vi "movimientocabinas.vi"() -> ()   [LabVIEW 2021]
panel:
  in  "BB 5":bool
  out "Graficas":cluster{"CabinaA":dbl, "CabinaB":dbl}(graph)
  in  "Demostrativa":bool
  in  "Colectiva":bool
  in  "Universal":bool
  out "Rele B":bool
  out "Rele A":bool
  out "Motor B":bool
  out "Motor A":bool
  out "fsb 5":bool
  out "fsb 4":bool
  out "fsb 3":bool
  out "fsb 2":bool
  out "fsa 5":bool
  out "fsa 3":bool
  out "fsa 4":bool
  out "fsa 2":bool
  in  "BB 4":bool
  out "LedB 4":bool
  in  "BB 3":bool
  out "LedB 3":bool
  in  "BB 2":bool
  out "LedB 2":bool
  in  "BB 1":bool
  out "LedB 1":bool
  out "LedB 5":bool
  in  "Cabina_B":dbl(slide) scale=1.0..5.0
  in  "BA 5":bool
  out "LedA 5":bool
  in  "BA 4":bool
  out "LedA 4":bool
  in  "BA 3":bool
  out "LedA 3":bool
  in  "BA 2":bool
  out "LedA 2":bool
  out "Display B":i32
  out "Display A":i32
  in  "Bit Restante B":bool
  in  "LSB B":bool
  in  "MSB B":bool
  in  "Bit Restante A":bool
  in  "LSB A":bool
  in  "MSB A":bool
  in  "BA 1":bool
  out "LedA 1":bool
  out "L_V":bool
  out "L_R":bool
  in  "Stop_PLC":bool
  in  "Start_PLC":bool
  out "fsb 1":bool
  out "fsa 1":bool
  in  "Tiempo_iteracion":u32
  in  "Baja B":bool
  in  "Cabina_A":dbl(slide) scale=1.0..5.0
  in  "Sube B":bool
  in  "Baja A":bool
  in  "Sube A":bool
  in  "STOP_LabVIEW":bool
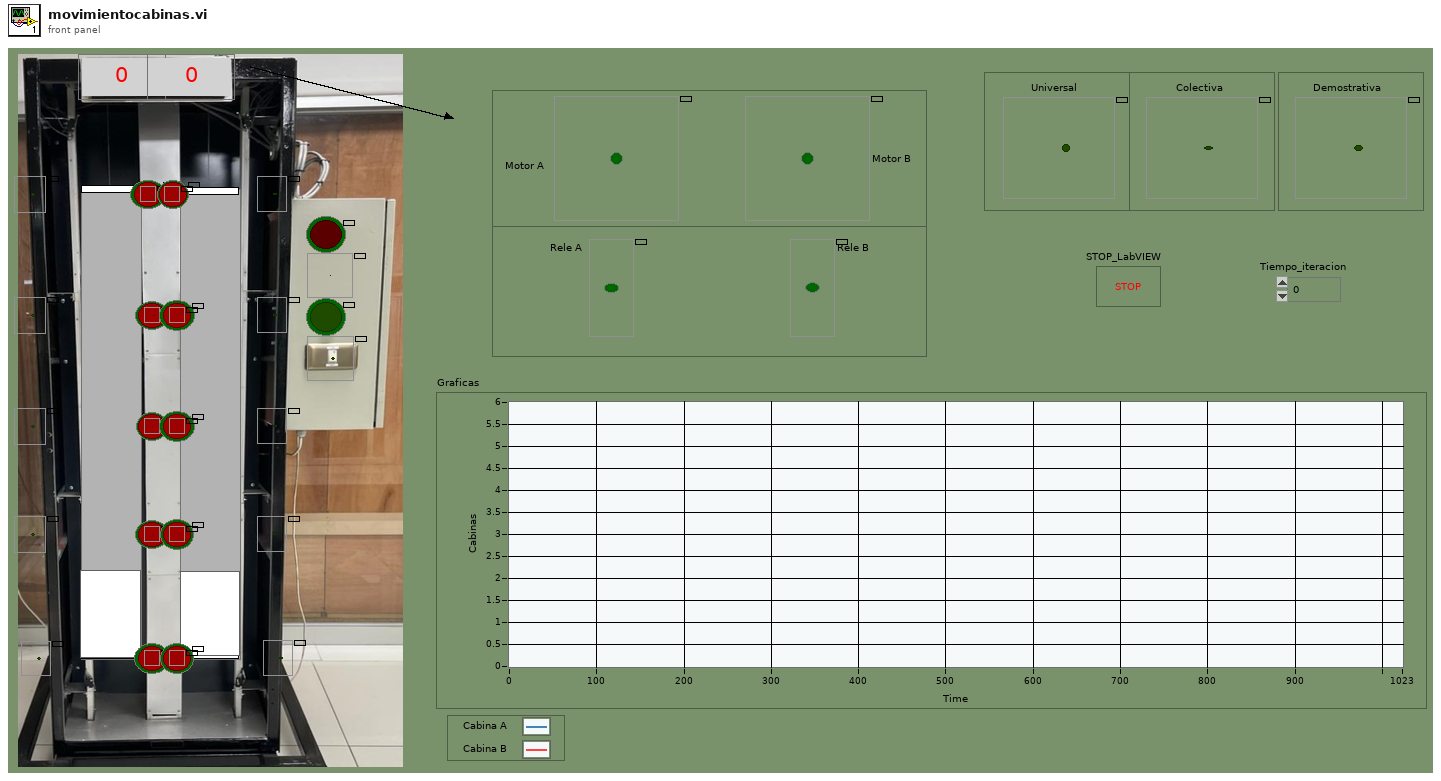
[diagram p1: front panel]
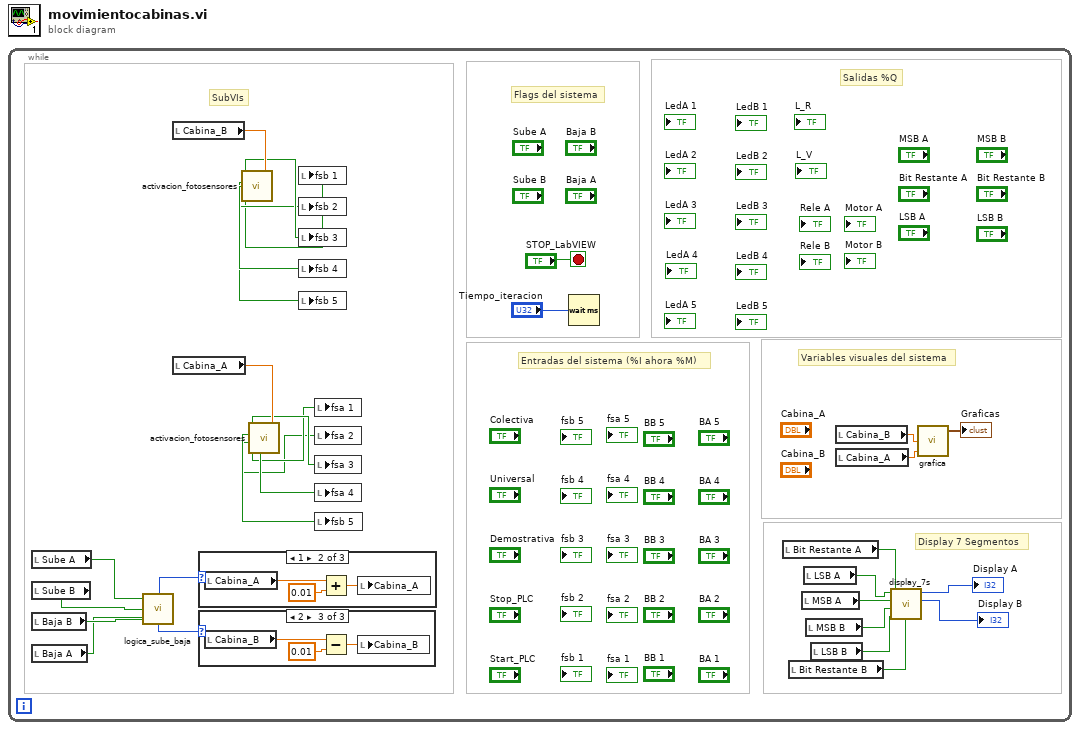
[diagram p0: block diagram]
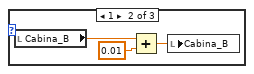
[diagram p3: hidden frame]
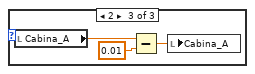
[diagram p5: hidden frame]
diagram:
  n1 = while {
    stop <- "STOP_LabVIEW" stop-if-true
    # "SubVIs"
    # "Entradas del sistema (%I ahora %M)"
    # "Variables visuales del sistema"
    # "Flags del sistema"
    # "Display 7 Segmentos"
    # "Salidas %Q"
    n2 = local read "Sube A"() -> (w16:bool)
    n3 = local read "Sube B"() -> (w15:bool)
    n4 = local read "Baja B"() -> (w14:bool)
    n5 = local read "Baja A"() -> (w13:bool)
    n6 = call "logica_sube_baja.vi"("Baja A"=w13, "Baja B"=w14, "Sube B"=w15, "Sube A"=w16) -> ("Numeric"=w29:i32, "Numeric 2"=w30:i32)
    n7 = local read "Cabina_B"() -> (w12:dbl)
    n8 = local read "Cabina_A"() -> (w11:dbl)
    n9 = case shown="1" w29 {
      frame 0, Default {
      }
      frame 1 {
        n10 = local read "Cabina_A"() -> (w39:dbl)
        n11 = Add(x=w39, y=0.01) -> (x+y=w40:dbl)
        n12 = local write "Cabina_A"(w40) -> ()
      }
      frame 2 {
        n13 = local read "Cabina_A"() -> (w42:dbl)
        n14 = Subtract(x=w42, y=0.01) -> (x-y=w41:dbl)
        n15 = local write "Cabina_A"(w41) -> ()
      }
    }
    n16 = case shown="2" w30 {
      frame 0, Default {
      }
      frame 1 {
        n17 = local read "Cabina_B"() -> (w34:dbl)
        n18 = Add(x=w34, y=0.01) -> (x+y=w33:dbl)
        n19 = local write "Cabina_B"(w33) -> ()
      }
      frame 2 {
        n20 = local read "Cabina_B"() -> (w36:dbl)
        n21 = Subtract(x=w36, y=0.01) -> (x-y=w37:dbl)
        n22 = local write "Cabina_B"(w37) -> ()
      }
    }
    n23 = call "activacion_fotosensores.vi"("Cabina"=w12) -> ("In Range? 3"=w4:bool, "In Range? 5"=w3:bool, "In Range? 2"=w2:bool, "In Range?"=w1:bool, "In Range? 4"=w5:bool)
    n24 = call "activacion_fotosensores.vi"("Cabina"=w11) -> ("In Range? 3"=w9:bool, "In Range? 5"=w8:bool, "In Range? 2"=w6:bool, "In Range?"=w7:bool, "In Range? 4"=w10:bool)
    n25 = local write "fsb 1"(w1) -> ()
    n26 = local write "fsb 2"(w2) -> ()
    n27 = local write "fsb 3"(w4) -> ()
    n28 = local write "fsb 4"(w5) -> ()
    n29 = local write "fsb 5"(w3) -> ()
    n30 = local write "fsa 1"(w7) -> ()
    n31 = local write "fsa 2"(w6) -> ()
    n32 = local write "fsa 3"(w9) -> ()
    n33 = local write "fsa 4"(w10) -> ()
    n34 = local write "fsb 5"(w8) -> ()
    n35 = Wait (ms)(milliseconds to wait="Tiempo_iteracion") -> ()  [unwired: 1 out]
    n36 = local read "Bit Restante A"() -> (w22:bool)
    n37 = local read "Bit Restante B"() -> (w17:bool)
    n38 = local read "MSB A"() -> (w20:bool)
    n39 = local read "LSB A"() -> (w21:bool)
    n40 = local read "MSB B"() -> (w19:bool)
    n41 = local read "LSB B"() -> (w18:bool)
    n42 = local read "Cabina_B"() -> (w27:dbl)
    n43 = local read "Cabina_A"() -> (w26:dbl)
    n44 = call "display_7s.vi"("Bit Restante B"=w17, "MSB A"=w20, "LSB B"=w18, "MSB B"=w19, "Bit Restante A"=w22, "LSB A"=w21) -> ("output variable 2"=→"Display B":i32, "output variable"=→"Display A":i32)
    n45 = call "grafica.vi"("CabinaA"=w26, "CabinaB"=w27) -> ("Graficas"=→"Graficas":cluster{"CabinaA":dbl, "CabinaB":dbl})
  }
